vi "QueryLakeshoreMeasurement (SubVI).vi"(8 "error in (no error)":errorcluster, 9 "Sample Channel Str":string, 10 "Cernox channel string":string, 11 "VISA Refnum in":refnum<visa-resource-name>) -> (0 "error out":errorcluster, 2 "Read output":string, 3 "VISA Refnum out":refnum<visa-resource-name>, 5 "Boolean":bool)   [LabVIEW 2017, in "Fridge Software v2.1.lvlib"]
uses:
  Fridge Software v2.1.lvlib
  <instrlib>/Lake Shore 372/Lake Shore 372.lvlib
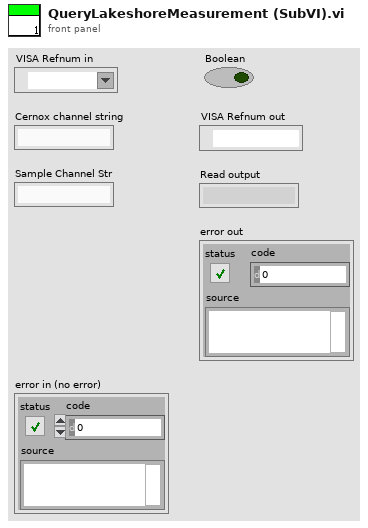
[diagram p1: front panel]
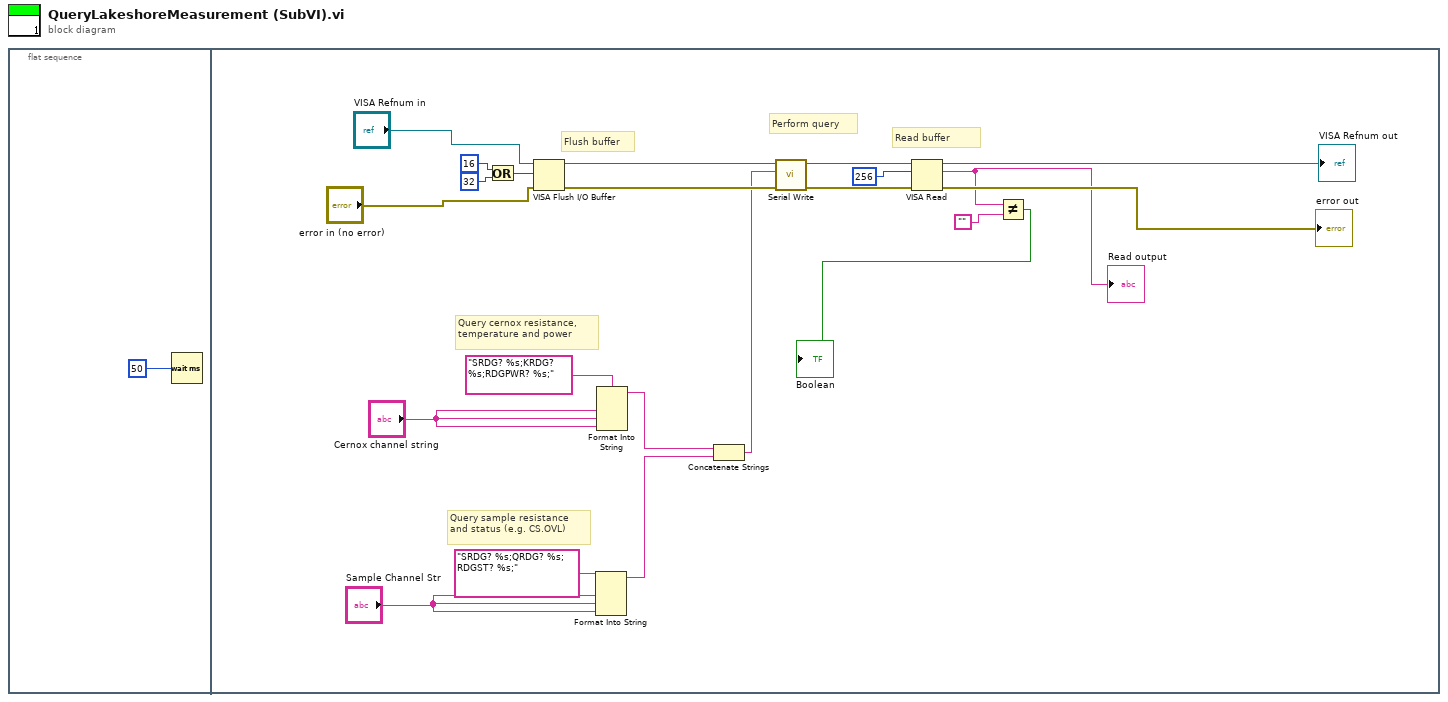
[diagram p0: block diagram]
diagram:
  n1 = flat-sequence {
    frame #0 {
      n2 = Wait (ms)(milliseconds to wait=50) -> ()  [unwired: 1 out]
    }
    frame #1 {
      # "Flush buffer"
      # "Query cernox resistance, temperature and power"
      # "Query sample resistance and status (e.g. CS.OVL)"
      # "Read buffer"
      # "Perform query"
      n3 = Or(x=16, y=32) -> (x .or. y?=w8:i32)
      n4 = VISA Flush I/O Buffer(VISA resource name="VISA Refnum in", mask (16)=w8, error in (no error)="error in (no error)") -> (VISA resource name out=w12:refnum<visa-resource-name>, error out=w21:errorcluster)
      n5 = Format Into String(format string="SRDG? %s;QRDG? %s; RDGST? %s;", "Sample Channel Str", "Sample Channel Str", "Sample Channel Str") -> (resulting string=w6:string)  [unwired: 2 in, 1 out]
      n6 = Format Into String(format string="SRDG? %s;KRDG? %s;RDGPWR? %s;", "Cernox channel string", "Cernox channel string", "Cernox channel string") -> (resulting string=w7:string)  [unwired: 2 in, 1 out]
      n7 = Concatenate Strings(w7, w6) -> (w20:string)
      n8 = call <instrlib>:"Serial Write.vi"("error in (no error)"=w21, "Write Buffer (\"\")"=w20, "VISA resource name"=w12) -> ("error out"=w22:errorcluster, "VISA resource name out"=w23:refnum<visa-resource-name>)  [unwired: 6 in, 1 out]
      n9 = VISA Read(VISA resource name=w23, byte count=u32 256, error in (no error)=w22) -> (VISA resource name out=→"VISA Refnum out":refnum<visa-resource-name>, read buffer=w15:string, error out=→"error out":errorcluster)  [unwired: 1 out]
      "Read output" <- w15
      n10 = Not Equal?(x=w15, y="") -> (x != y?=→"Boolean":bool)
    }
  }
